vi "DIO Read.vi"(2 "Channels":i32[](array[numeric]), 3 "device":i16=1) -> (0 "Error":bool, 1 "Data":bool[](array[boolean]))   [LabVIEW 2019]
uses:
  <vilib>/DAQmx/read.llb/DAQmx Read (Digital 1D Bool 1Chan 1Samp).vi
  <vilib>/DAQmx/create/channels.llb/DAQmx Create Channel (DI-Digital Input).vi
  <vilib>/DAQmx/miscellaneous.llb/DAQmx Fill In Error Info.vi
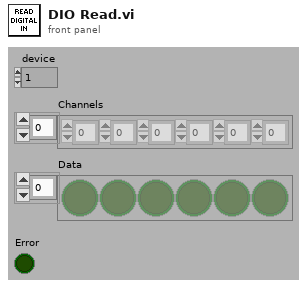
[diagram p1: front panel]
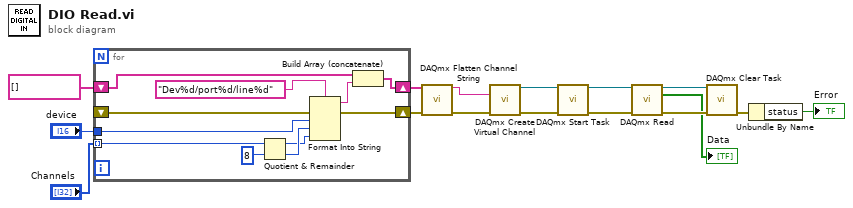
[diagram p0: block diagram]
diagram:
  n1 = for {
    tunnel: "Channels" -> [w23] mode=indexing
    tunnel: "device" -> [w24]
    shift-right: [w27] -> w13
    shift-left: tag[] [] -> [w26]
    shift-right: [w19] -> w1
    shift-left: _ -> [w18]
    n2 = Quotient & Remainder(x=w23, y=8) -> (x-y*floor(x/y)=w20:i32, floor(x/y)=w21:i32)
    n3 = Format Into String(format string="Dev%d/port%d/line%d", error in=w18, w24, w21, w20) -> (resulting string=w17:string, error out=w19:errorcluster)  [unwired: 1 in]
    n4 = Build Array (concatenate)(w26, w17) -> (w27:string[])
  }
  n5 = call <vilib>:"DAQmx Flatten Channel String.vi"("names in"=w13, "error in"=w1) -> ("names out"=w12:string, "error out"=w14:errorcluster)  [unwired: 12 in]
  n6 = call-poly <vilib>:"DAQmx Create Virtual Channel.vi"("lines"=w12, "error in"=w14) -> ("task out"=w11:refnum<k21>, "error out"=w10:errorcluster)  [unwired: 12 in]
  n7 = call <vilib>:"DAQmx Start Task.vi"("task/channels in"=w11, "error in"=w10) -> ("task out"=w9:refnum<k21>, "error out"=w8:errorcluster)  [unwired: 12 in]
  n8 = call-poly <vilib>:"DAQmx Read.vi"("task/channels in"=w9, "error in"=w8) -> ("task out"=w7:refnum<k21>, "data"=→"Data":bool[], "error out"=w6:errorcluster)  [unwired: 11 in]
  n9 = call <vilib>:"DAQmx Clear Task.vi"("task in"=w7, "error in"=w6) -> ("error out"=w5:errorcluster)  [unwired: 13 in]
  n10 = Unbundle By Name(w5) -> ("status"=→"Error":bool)
